vi "Grid Activate.vi"(8 "error in (no error)":errorcluster, 11 "SCADA in":refnum<class "SCADA.lvclass">) -> (0 "error out":errorcluster, 3 "SCADA out":refnum<class "SCADA.lvclass">)   [LabVIEW 2015, in "SCADA Core.lvlib" / "SCADA.lvclass"]
uses:
  SCADA.lvclass
  IED Actor/IED/Controls/Device Activate Mode Select.ctl
  <vilib>/ActorFramework/Actor/Actor.lvclass/Actor.ctl
  <vilib>/ActorFramework/Message Enqueuer/Message Enqueuer.lvclass/Message Enqueuer.ctl
  SCADA.lvclass/SCADA.ctl
  SCADA Messages/Set Number of Activations Msg/Set Number of Activations Msg.lvclass/Set Number of Activations Msg.ctl
  Controls/Queue Selector.ctl
  IED Actor/IED Messages/Device Activate Msg/Device Activate Msg.lvclass/Device Activate Msg.ctl
  Controls/Grid Mode.ctl
  <vilib>/ActorFramework/Message Enqueuer/Init from Existing Queue.vi
  <vilib>/ActorFramework/Message Enqueuer/Enqueue.vi
  <vilib>/ActorFramework/Message Priority Queue/Priority Enqueue.vi
  <vilib>/ActorFramework/Message Enqueuer/Message Enqueuer.lvclass
  SCADA Messages/Set Number of Activations Msg/Set Number of Activations Msg.lvclass
  IED Actor/IED Messages/Device Activate Msg/Device Activate Msg.lvclass
  <vilib>/ActorFramework/Actor/Actor.lvclass
  IED Actor/IED/IED.lvclass
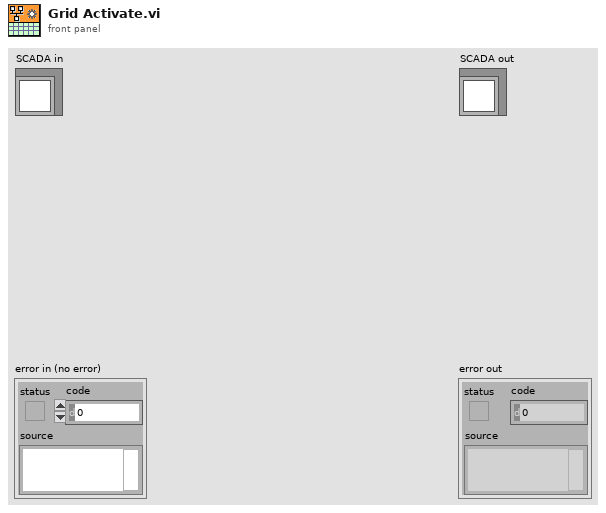
[diagram p1: front panel]
types:
  T1 = typedef "SCADA Core.lvlib/SCADA.lvclass/Grid Mode.ctl" = enum16{"Off", "Grid Connected", "Islanded", "Synchronizing"}
  T2 = typedef "SCADA Core.lvlib/SCADA.lvclass/Queue Selector.ctl" = enum16{"IEDs", "PV", "Generators", "Wind", "Storage", "Relays"}
  T3 = typedef "IED Actor.lvlib/IED.lvclass/Device Activate Mode Select.ctl" = enum16{"Activate", "Blackstart", "Individual"}
  T4 = typedef "Tools_KeyedArray.lvlib/KeyedArray.ctl" = cluster{"keys":string[], "values":string[]}
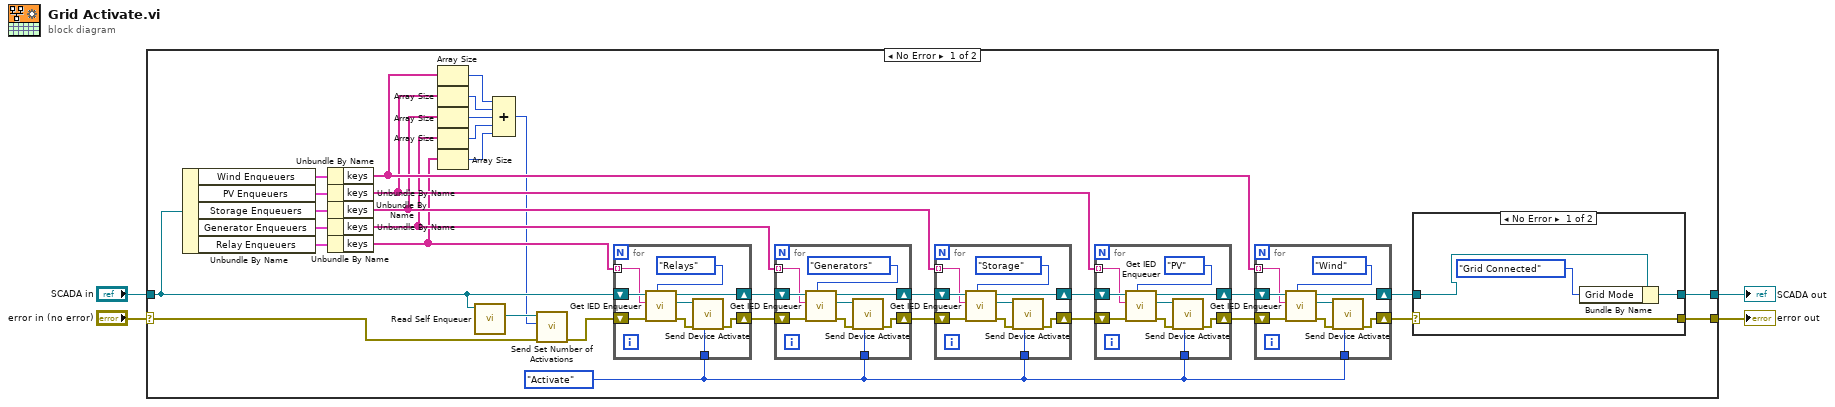
[diagram p0: block diagram]
diagram:
  n1 = case shown="No Error" "error in (no error)" {
    selector: "error in (no error)" -> [w14 w90]
    tunnel: [w8 w90] -> w3
    tunnel: [w7 w89] -> w1
    tunnel: "SCADA in" -> [w12 w89]
    frame No Error {
      w5 = Device_Activate_Mode_Select."Activate" ("Activate Mode")
      n2 = Unbundle By Name(w12) -> ("Wind Enqueuers"=w28:T4, "PV Enqueuers"=w27:T4, "Storage Enqueuers"=w26:T4, "Generator Enqueuers"=w25:T4, "Relay Enqueuers"=w29:T4)
      n3 = Unbundle By Name(w28) -> ("keys"=w19:string[])
      n4 = Unbundle By Name(w27) -> ("keys"=w18:string[])
      n5 = Unbundle By Name(w26) -> ("keys"=w17:string[])
      n6 = Unbundle By Name(w25) -> ("keys"=w16:string[])
      n7 = Unbundle By Name(w29) -> ("keys"=w15:string[])
      n8 = Array Size(array=w19) -> (size(s)=w24:i32)
      n9 = Array Size(array=w18) -> (size(s)=w23:i32)
      n10 = Array Size(array=w17) -> (size(s)=w22:i32)
      n11 = Array Size(array=w16) -> (size(s)=w21:i32)
      n12 = Array Size(array=w15) -> (size(s)=w20:i32)
      n13 = call <vilib>:"Read Self Enqueuer.vi"("Actor"=w12) -> ("Self Enqueuer"=w11:refnum<class "Message Enqueuer.lvclass">)  [unwired: 10 in]
      n14 = Compound Arithmetic op=ADD(w24, w23, w22, w21, w20) -> (w10:i32)
      n15 = call "Send Set Number of Activations.vi"("error in (no error)"=w14, "Number of Activations"=w10, "Message Enqueuer"=w11) -> ("error out"=w13:errorcluster)  [unwired: 7 in, 1 out]
      n16 = for {
        shift-right: [w83] -> w37
        shift-left: w13 -> [w87]
        tunnel: w15 -> [w86] mode=indexing
        shift-right: [w82] -> w33
        shift-left: w12 -> [w88]
        tunnel: w5 -> [w80]
        n17 = call "Get IED Enqueuer.vi"("Queue (IEDs)"=Queue_Selector."Relays" ("Queue"), "error in (no error)"=w87, "IED Name"=w86, "SCADA in"=w88) -> ("error out"=w85:errorcluster, "IED Enqueuer"=w84:refnum<class "Message Enqueuer.lvclass">, "SCADA out"=w82:refnum<class "SCADA.lvclass">)  [unwired: 5 in]
        n18 = call "Send Device Activate.vi"("Activate Mode"=w80, "error in (no error)"=w85, "Message Enqueuer"=w84) -> ("error out"=w83:errorcluster)  [unwired: 7 in, 1 out]
      }
      n19 = for {
        shift-right: [w74] -> w36
        shift-left: w37 -> [w78]
        tunnel: w16 -> [w77] mode=indexing
        shift-right: [w73] -> w32
        shift-left: w33 -> [w79]
        tunnel: w5 -> [w71]
        n20 = call "Get IED Enqueuer.vi"("Queue (IEDs)"=Queue_Selector."Generators" ("Queue"), "error in (no error)"=w78, "IED Name"=w77, "SCADA in"=w79) -> ("error out"=w76:errorcluster, "IED Enqueuer"=w75:refnum<class "Message Enqueuer.lvclass">, "SCADA out"=w73:refnum<class "SCADA.lvclass">)  [unwired: 5 in]
        n21 = call "Send Device Activate.vi"("Activate Mode"=w71, "error in (no error)"=w76, "Message Enqueuer"=w75) -> ("error out"=w74:errorcluster)  [unwired: 7 in, 1 out]
      }
      n22 = for {
        shift-right: [w65] -> w35
        shift-left: w36 -> [w69]
        tunnel: w17 -> [w68] mode=indexing
        shift-right: [w64] -> w31
        shift-left: w32 -> [w70]
        tunnel: w5 -> [w62]
        n23 = call "Get IED Enqueuer.vi"("Queue (IEDs)"=Queue_Selector."Storage" ("Queue"), "error in (no error)"=w69, "IED Name"=w68, "SCADA in"=w70) -> ("error out"=w67:errorcluster, "IED Enqueuer"=w66:refnum<class "Message Enqueuer.lvclass">, "SCADA out"=w64:refnum<class "SCADA.lvclass">)  [unwired: 5 in]
        n24 = call "Send Device Activate.vi"("Activate Mode"=w62, "error in (no error)"=w67, "Message Enqueuer"=w66) -> ("error out"=w65:errorcluster)  [unwired: 7 in, 1 out]
      }
      n25 = for {
        shift-right: [w56] -> w34
        shift-left: w35 -> [w60]
        tunnel: w18 -> [w59] mode=indexing
        shift-right: [w55] -> w30
        shift-left: w31 -> [w61]
        tunnel: w5 -> [w53]
        n26 = call "Get IED Enqueuer.vi"("Queue (IEDs)"=Queue_Selector."PV" ("Queue"), "error in (no error)"=w60, "IED Name"=w59, "SCADA in"=w61) -> ("error out"=w58:errorcluster, "IED Enqueuer"=w57:refnum<class "Message Enqueuer.lvclass">, "SCADA out"=w55:refnum<class "SCADA.lvclass">)  [unwired: 5 in]
        n27 = call "Send Device Activate.vi"("Activate Mode"=w53, "error in (no error)"=w58, "Message Enqueuer"=w57) -> ("error out"=w56:errorcluster)  [unwired: 7 in, 1 out]
      }
      n28 = for {
        shift-right: [w47] -> w9
        shift-left: w34 -> [w51]
        tunnel: w19 -> [w50] mode=indexing
        shift-right: [w46] -> w6
        shift-left: w30 -> [w52]
        tunnel: w5 -> [w44]
        n29 = call "Get IED Enqueuer.vi"("Queue (IEDs)"=Queue_Selector."Wind" ("Queue"), "error in (no error)"=w51, "IED Name"=w50, "SCADA in"=w52) -> ("error out"=w49:errorcluster, "IED Enqueuer"=w48:refnum<class "Message Enqueuer.lvclass">, "SCADA out"=w46:refnum<class "SCADA.lvclass">)  [unwired: 5 in]
        n30 = call "Send Device Activate.vi"("Activate Mode"=w44, "error in (no error)"=w49, "Message Enqueuer"=w48) -> ("error out"=w47:errorcluster)  [unwired: 7 in, 1 out]
      }
      n31 = case shown="No Error" w9 {
        selector: w9 -> [w41 w43]
        tunnel: [w41 w43] -> w8
        tunnel: [w39 w42] -> w7
        tunnel: w6 -> [w40 w42]
        frame No Error {
          n32 = Bundle By Name(cluster=w40, "Grid Mode"=Grid_Mode."Grid Connected") -> (w39:refnum<class "SCADA.lvclass">)
        }
        frame Error {
        }
      }
    }
    frame Error {
    }
  }
  "error out" <- w3
  "SCADA out" <- w1
